vi "Timeout_Delay.vi"   [LabVIEW 2014]
uses:
  <vilib>/Aledyne-TSXperts/Arduino Compatible Compiler for LabVIEW/Code Generator/Arduino APIs/Digital/PinDirection.ctl
  QwaveSys_ESP8266/QwaveSys_ESP8266.lvlib
  <vilib>/Aledyne-TSXperts/Arduino Compatible Compiler for LabVIEW/Arduino Compatible Compiler for LabVIEW.lvlib
types:
  T1 = typedef "Arduino Compatible Compiler for LabVIEW.lvlib/PinDirection.ctl" = enum16{" INPUT", "OUTPUT", " INPUT_PULLUP"}
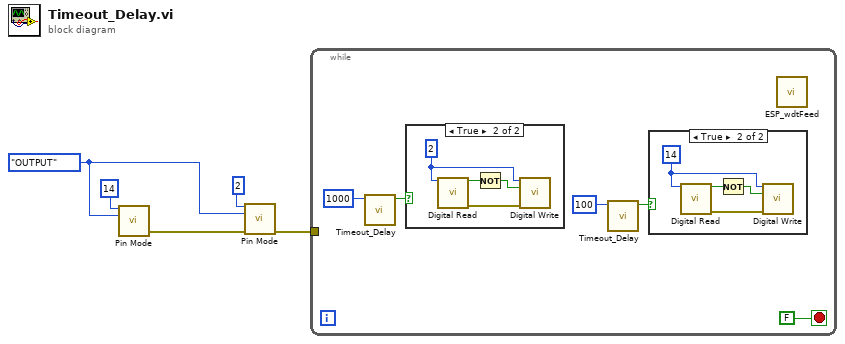
[diagram p0: block diagram]
diagram:
  w3 = PinDirection."OUTPUT" ("direction")
  n1 = call <vilib>:"Pin Mode.vi"("pin"=u8 14, "direction"=w3) -> ("error out"=w2:errorcluster)  [unwired: 13 in]
  n2 = call <vilib>:"Pin Mode.vi"("pin"=u8 2, "direction"=w3, "error in (no error)"=w2) -> ("error out"=w1:errorcluster)  [unwired: 12 in]
  n3 = while {
    tunnel: w1 -> [_]
    stop <- FALSE stop-if-true
    n4 = call "Timeout_Delay.vi"("timeout (ms)"=u32 1000) -> ("status"=w8:bool)  [unwired: 8 in, 2 out]
    n5 = case shown="True" w8 {
      frame False {
      }
      frame True {
        w16 = u8 2 ("pin")
        n6 = call <vilib>:"Digital Read.vi"("pin"=w16) -> ("state"=w18:bool, "error out"=w15:errorcluster)  [unwired: 13 in]
        n7 = Not(x=w18) -> (.not. x?=w17:bool)
        n8 = call <vilib>:"Digital Write.vi"("pin"=w16, "state"=w17, "error in (no error)"=w15) -> ()  [unwired: 12 in, 1 out]
      }
    }
    n9 = call "Timeout_Delay.vi"("timeout (ms)"=u32 100) -> ("status"=w7:bool)  [unwired: 8 in, 2 out]
    n10 = case shown="True" w7 {
      frame False {
      }
      frame True {
        w12 = u8 14 ("pin")
        n11 = call <vilib>:"Digital Read.vi"("pin"=w12) -> ("state"=w14:bool, "error out"=w11:errorcluster)  [unwired: 13 in]
        n12 = Not(x=w14) -> (.not. x?=w13:bool)
        n13 = call <vilib>:"Digital Write.vi"("pin"=w12, "state"=w13, "error in (no error)"=w11) -> ()  [unwired: 12 in, 1 out]
      }
    }
    n14 = call "ESP_wdtFeed.vi"() -> ()  [unwired: 11 in, 1 out]
  }
